vi "Main.vi"() -> ()   [LabVIEW 2016]
doc: "The myRIO Project template acquires acceleration data from the onboard accelerometer and displays the changes of acceleration values in a waveform chart."
uses:
  040-typeDefs/Position.ctl
  <vilib>/myRIO/Common/Instrument Driver Framework/myRIO v1.0/Encoder/typedefs/Encoder Signal Mode.ctl
  <vilib>/myRIO/Instrument Drivers/Onboard IO/Encoder/typedefs/Encoder Reference.ctl
  <vilib>/myRIO/Common/Instrument Driver Framework/Utilities/typedefs/myRIO Generic Hardware Reference.ctl
  <vilib>/myRIO/Common/Instrument Driver Framework/Utilities/typedefs/Hardware Version Enum.ctl
  <vilib>/myRIO/Common/Instrument Driver Framework/Utilities/typedefs/myRIO v1.0 Reference.ctl
  <vilib>/myRIO/Common/Instrument Driver Framework/Utilities/typedefs/Generic FPGA Reference.ctl
  <vilib>/myRIO/Common/Instrument Driver Framework/myRIO v1.0/Encoder/typedefs/Encoder Channels Enum.ctl
  <vilib>/myRIO/Common/Instrument Driver Framework/myRIO v1.0/Encoder/typedefs/Encoder Configuration v1.0.ctl
  <vilib>/userdefined/High Color/nirio_resource_hc.ctl
  <vilib>/myRIO/Instrument Drivers/Onboard IO/PWM/typedefs/PWM Reference.ctl
  <vilib>/myRIO/Common/Instrument Driver Framework/myRIO v1.0/PWM/typedefs/PWM Channels Enum.ctl
  <vilib>/myRIO/Instrument Drivers/Onboard IO/PWM/typedefs/PWM Configuration.ctl
  <vilib>/myRIO/Common/Instrument Driver Framework/Utilities/vis/Is FPGA Ref Available.vi
  <vilib>/myRIO/Common/Instrument Driver Framework/myRIO v1.0/Encoder/vis/myRIO v1.1 Open Encoder.vi
  <vilib>/myRIO/Instrument Drivers/Onboard IO/Encoder/vis/Read.vi
  <vilib>/myRIO/Common/Instrument Driver Framework/myRIO v1.0/PWM/vis/myRIO v1.1 Open PWM.vi
  <vilib>/myRIO/Instrument Drivers/Onboard IO/PWM/vis/Set Duty Cycle and Frequency.vi
  <vilib>/myRIO/Common/Instrument Driver Framework/Utilities/vis/Validate Channels.vi
  <vilib>/myRIO/Common/Instrument Driver Framework/myRIO v1.0/Encoder/vis/myRIO v1.0 Reserve Encoder.vi
  <vilib>/myRIO/Common/Instrument Driver Framework/myRIO v1.0/PWM/vis/myRIO v1.0 Reserve PWM.vi
  <vilib>/myRIO/Common/Instrument Driver Framework/myRIO v1.0/Encoder/vis/myRIO v1.0 Build MUX Configuration Encoder.vi
  <vilib>/myRIO/Common/Instrument Driver Framework/myRIO v1.0/Resource Manager/vis/myRIO v1.0 Reserve Channel List.vi
  <vilib>/myRIO/Common/Instrument Driver Framework/myRIO v1.0/PWM/vis/myRIO v1.0 Build MUX Configuration PWM.vi
  <vilib>/myRIO/Common/Instrument Driver Framework/myRIO v1.0/Resource Manager/vis/myRIO v1.0 Create Configuration List.vi
  <vilib>/myRIO/Common/Instrument Driver Framework/myRIO v1.0/Resource Manager/vis/myRIO v1.0 Reserve Channel.vi
  <vilib>/myRIO/Common/Instrument Driver Framework/myRIO v1.0/Resource Manager/vis/myRIO v1.0 Unreserve Channel.vi
  <vilib>/myRIO/Common/Instrument Driver Framework/myRIO v1.0/Resource Manager/vis/myRIO v1.0 Build Mutex Name.vi
  <vilib>/Utility/VariantDataType/GetNumericInfo.vi
  <vilib>/Utility/error.llb/Error Cluster From Error Code.vi
  <vilib>/myRIO/Common/Instrument Driver Framework/myRIO v1.0/myRIO v1.1 Open.vi
  <vilib>/myRIO/Common/Instrument Driver Framework/Utilities/vis/IO Manager.vi
  <vilib>/myRIO/Common/Instrument Driver Framework/Utilities/vis/Configuration Manager.vi
  <vilib>/myRIO/Common/Instrument Driver Framework/myRIO v1.0/Resource Manager/vis/myRIO v1.0 Configure IO.vi
  <vilib>/myRIO/Common/Instrument Driver Framework/myRIO v1.0/myRIO v1.0 Close.vi
  <vilib>/myRIO/Common/Instrument Driver Framework/myRIO v1.0/Encoder/vis/myRIO v1.0 Configure Encoder.vi
  <vilib>/myRIO/Common/Instrument Driver Framework/myRIO v1.0/Encoder/vis/myRIO v1.0 Read Encoder.vi
  <vilib>/myRIO/Common/Instrument Driver Framework/myRIO v1.0/PWM/vis/myRIO v1.0 Write PWM.vi
  <vilib>/myRIO/Express VI/Onboard IO/Encoder/Encoder Express VI.xnode
  <vilib>/myRIO/Instrument Drivers/Onboard IO/Encoder/vis/myRIO Encoder Open.xnode
  <vilib>/myRIO/Express VI/Onboard IO/PWM/PWM Express VI.xnode
  <vilib>/myRIO/Instrument Drivers/Onboard IO/PWM/vis/myRIO PWM Open.xnode
  <vilib>/myRIO/Instrument Drivers/Onboard IO/Encoder/Encoder.lvlib
  <vilib>/myRIO/Instrument Drivers/Onboard IO/PWM/PWM.lvlib
panel:
  in  "PID":bool
  in  "Map":bool
  in  "Odometry":bool
  in  "Main":bool
  out "Odometery":T1
  out "?":cluster{dbl[], dbl[]}(graph)
  in  "?":T1
  in  "Motor Gear Ratio":dbl
  in  "Encoder Ticks/Rev":dbl
  in  "Wheel Diameter":dbl
  in  "Wheel Base Length":dbl
  out "Speed B":dbl
  out "Speed A":dbl
  out "EncoderB Diff":i32
  out "EncoderA Diff":i32
  # "Robot Odometry"
  # "Inital Position"
  # "Enable/Disable Loop"
  # "NIARC 2018 UNSW"
  # "Robot Settings"
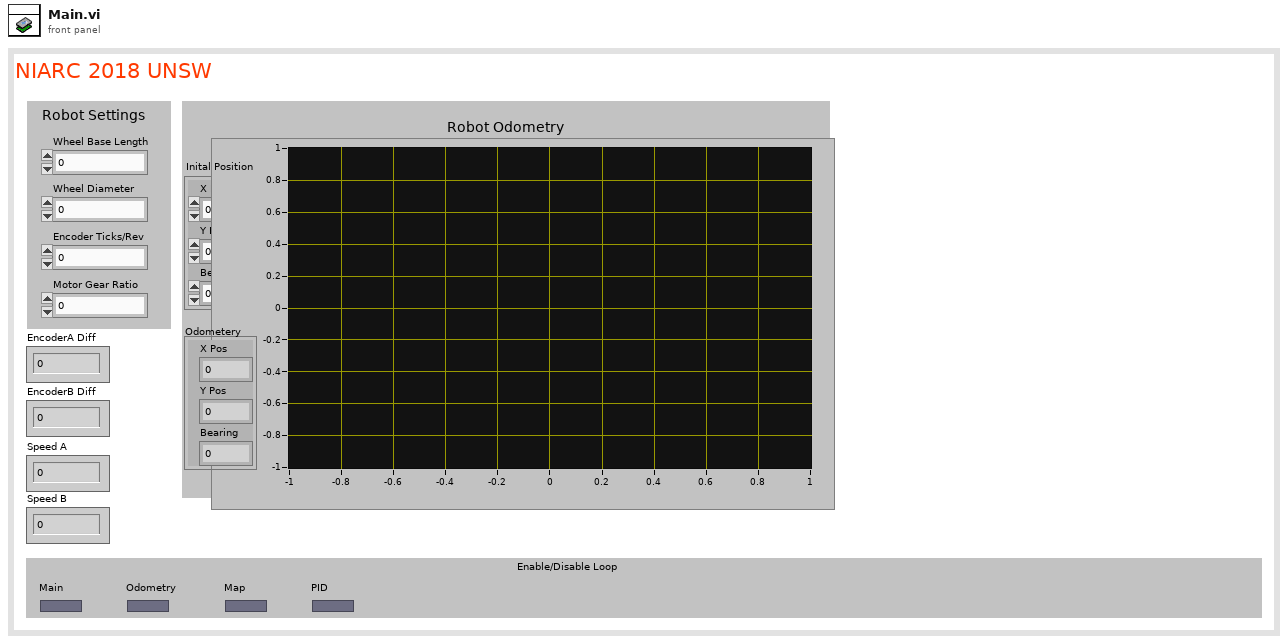
[diagram p1: front panel]
types:
  T1 = typedef "Position.ctl" = cluster{"X Pos":dbl, "Y Pos":dbl, "Bearing":dbl}
  T2 = typedef "Encoder.lvlib/Encoder Reference.ctl" = cluster{"myRIO Reference":T3, "Encoder Channels Enum":T7}
  T3 = typedef "myRIO Generic Hardware Reference.ctl" = cluster{"myRIO Model":T4, "myRIO Hardware Reference":T5}
  T4 = typedef "Hardware Version Enum.ctl" = enum16{"Unknown", "myRIO-1900", "myRIO-1950", "roboRIO", "NI ELVIS RIO CM"}
  T5 = typedef "myRIO v1.0 Reference.ctl" = cluster{"Generic FPGA Reference":T6, "Allow multiple opens":bool}
  T6 = typedef "Generic FPGA Reference.ctl" = refnum<k20>
  T7 = typedef "Encoder Channels Enum.ctl" = enum16{"Not Connected", "C/ENC0", "C/ENC1", "A/ENC", "B/ENC", "DIO/ENC0", "DIO/ENC1", "DIO/ENC2", "DIO/ENC3", "DIO/ENC4"}
  T8 = typedef "Encoder Signal Mode.ctl" = enum16{"Quadrature phase signal", "Step and direction signal"}
  T9 = typedef "nirio_resource_hc.ctl" = tag
  T10 = typedef "PWM.lvlib/PWM Reference.ctl" = cluster{"myRIO Reference":T3, "PWM Channels Enum":T11, "PWM Configuration":T12}
  T11 = typedef "PWM Channels Enum.ctl" = enum16{"Not Connected", "C/PWM0", "C/PWM1", "A/PWM0", "A/PWM1", "A/PWM2", "B/PWM0", "B/PWM1", "B/PWM2", "PWM/PWM0", "PWM/PWM1", "PWM/PWM2", "PWM/PWM3", "PWM/PWM4", "PWM/PWM5", "PWM/PWM6", "PWM/PWM7", "PWM/PWM8", "PWM/PWM9"}
  T12 = typedef "PWM.lvlib/PWM Configuration.ctl" = cluster{"Frequency":dbl, "Duty Cycle":dbl}
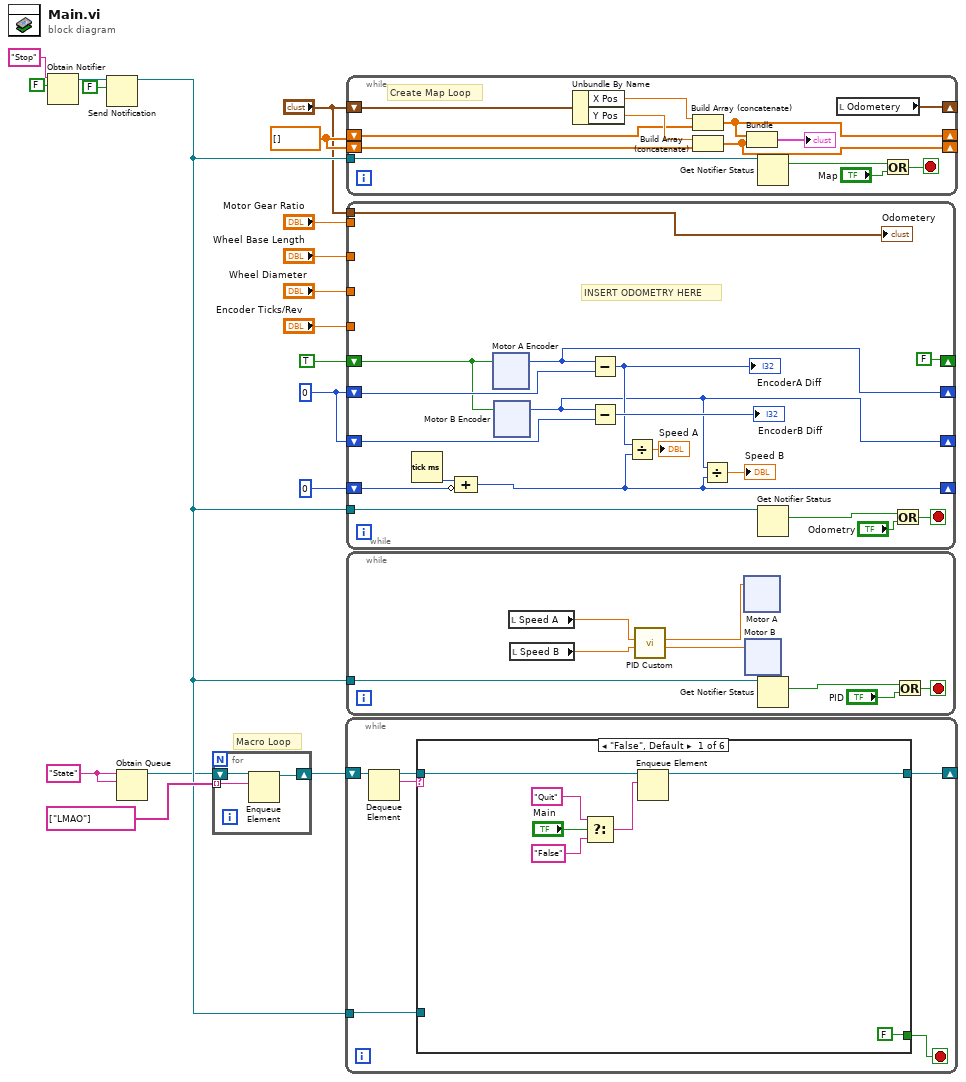
[diagram p0: block diagram]
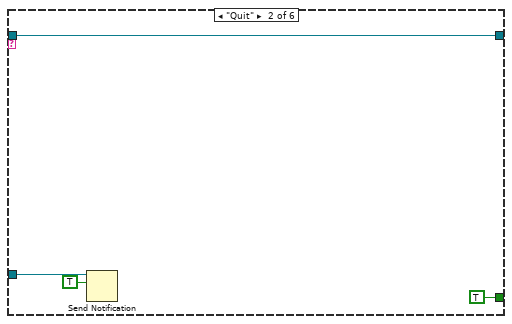
[diagram p2: hidden frame]
diagram:
  w1 = "State" ("name (unnamed)")
  w6 = dbl[] []
  w15 = 0
  # "Macro Loop"
  n1 = Obtain Notifier(name (unnamed)="Stop", notification data type=FALSE) -> (notifier out=w17:refnum<notifier>)  [unwired: 2 in, 2 out]
  n2 = Send Notification(notification=FALSE, notifier=w17) -> (notifier out=w7:refnum<notifier>)  [unwired: 1 in, 1 out]
  n3 = Obtain Queue(name (unnamed)=w1, element data type=w1) -> (queue out=w4:refnum<queue>)  [unwired: 3 in, 2 out]
  n4 = for {
    tunnel: string[] ["LMAO"] -> [w19] mode=indexing
    shift-right: [w21] -> w2
    shift-left: w4 -> [w20]
    n5 = Enqueue Element(queue=w20, element=w19) -> (queue out=w21:refnum<queue>)  [unwired: 2 in, 2 out]
  }
  n6 = while {
    shift-right: [w27] -> _
    shift-left: w2 -> [w23]
    tunnel: w7 -> [w25]
    stop <- w26 stop-if-true
    n7 = Dequeue Element(queue=w23) -> (queue out=w24:refnum<queue>, element=w22:string)  [unwired: 2 in, 2 out]
    n8 = case shown="\"False\", Default" w22 {
      tunnel: w24 -> [w34 w38 w39 w40 w41 w42]
      tunnel: [w33 w38 w39 w40 w41 w42] -> w27
      tunnel: [FALSE TRUE _ _ _ _] -> w26
      tunnel: w25 -> [_ w36 _ _ _ _]
      frame "False", Default {
        n9 = Select(t="Quit" ("element"), s="Main", f="False" ("element")) -> (s? t:f=w28:string)
        n10 = Enqueue Element(queue=w34, element=w28) -> (queue out=w33:refnum<queue>)  [unwired: 2 in, 2 out]
      }
      frame "Quit" {
        n11 = Send Notification(notification=TRUE, notifier=w36) -> ()  [unwired: 1 in, 2 out]
      }
      frame "Localise" {
      }
      frame "Path Plan" {
      }
      frame "Obstacle" {
      }
      frame "Wall Follow" {
      }
    }
  }
  n12 = while {
    tunnel: w7 -> [w55]
    shift-right: [w49] -> _
    shift-left: w6 -> [w51]
    shift-right: [w48] -> _
    shift-left: w6 -> [w47]
    shift-right: [w46] -> _
    shift-left: "?" -> [w53]
    stop <- w45 stop-if-true
    # "Create Map Loop"
    n13 = Unbundle By Name(w53) -> ("X Pos"=w50:dbl, "Y Pos"=w52:dbl)
    n14 = Build Array (concatenate)(w50, w51) -> (w49:dbl[])
    n15 = Build Array (concatenate)(w52, w47) -> (w48:dbl[])
    n16 = Bundle(w49, w48) -> (→"?":cluster{dbl[], dbl[]})  [unwired: 1 in]
    n17 = Get Notifier Status(notifier=w55) -> (current notification=w43:bool)  [unwired: 1 in, 4 out]
    n18 = local read "Odometery"() -> (w46:T1)
    n19 = Or(x=w43, y="Map") -> (x .or. y?=w45:bool)
  }
  n20 = while {
    tunnel: w7 -> [w73]
    shift-right: [w71] -> _
    shift-left: w15 -> [w72]
    shift-right: [w63] -> _
    shift-left: w15 -> [w70]
    shift-right: [FALSE] -> _
    shift-left: TRUE -> [w68]
    shift-right: [w62] -> _
    shift-left: 0 -> [w65]
    tunnel: "Motor Gear Ratio" -> [_]
    tunnel: "Wheel Base Length" -> [_]
    tunnel: "Wheel Diameter" -> [_]
    tunnel: "Encoder Ticks/Rev" -> [_]
    tunnel: "?" -> [w59]
    stop <- w57 stop-if-true
    # "INSERT ODOMETRY HERE"
    n21 = Tick Count (ms)() -> (millisecond timer value=w66:u32)
    n22 = Compound Arithmetic op=ADD(w66, invert w65) -> (w62:u32)
    n23 = xnode "Motor A Encoder"("Reset Counter"=w68) -> ("Counter Value"=w71:i32)  [unwired: 1 in, 3 out]
    n24 = xnode "Motor B Encoder"("Reset Counter"=w68) -> ("Counter Value"=w63:i32)  [unwired: 1 in, 3 out]
    n25 = Subtract(x=w71, y=w72) -> (x-y=w64:i32)
    "EncoderA Diff" <- w64
    n26 = Subtract(x=w63, y=w70) -> (x-y=→"EncoderB Diff":i32)
    n27 = Divide(x=w64, y=w62) -> (x/y=→"Speed A":dbl)
    n28 = Divide(x=w63, y=w62) -> (x/y=→"Speed B":dbl)
    n29 = Get Notifier Status(notifier=w73) -> (current notification=w58:bool)  [unwired: 1 in, 4 out]
    n30 = Or(x=w58, y="Odometry") -> (x .or. y?=w57:bool)
    "Odometery" <- w59
  }
  n31 = while {
    tunnel: w7 -> [w169]
    stop <- w168 stop-if-true
    n32 = local read "Speed A"() -> (w173:dbl)
    n33 = local read "Speed B"() -> (w172:dbl)
    n34 = call "PID Custom.vi"("Error Motor B"=w172, "Error Motor A"=w173) -> ("Output 2"=w170:dbl, "Output"=w171:dbl)  [unwired: 7 in, 1 out]
    n35 = xnode "Motor A"("Duty Cycle"=w171) -> ()  [unwired: 1 in, 1 out]
    n36 = xnode "Motor B"("Duty Cycle"=w170) -> ()  [unwired: 1 in, 1 out]
    n37 = Get Notifier Status(notifier=w169) -> (current notification=w166:bool)  [unwired: 1 in, 4 out]
    n38 = Or(x=w166, y="PID") -> (x .or. y?=w168:bool)
  }
